vi "Probe.vi"(8 "error in (no error)":errorcluster, 10 "Buffer":u8[](array[numeric]), 11 "Raw Message in":refnum<class "Raw Message.lvclass">) -> (0 "error out":errorcluster, 1 "Valid":bool, 2 "Buffer Count":i32, 3 "Raw Message out":refnum<class "Raw Message.lvclass">)   [LabVIEW 2020, in "Protobuf RAW.lvlib" / "Raw Message.lvclass"]
uses:
  Raw Message.lvclass
  Raw Message.lvclass/Raw Message.ctl
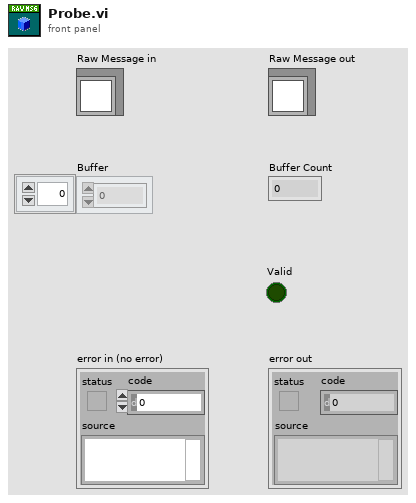
[diagram p1: front panel]
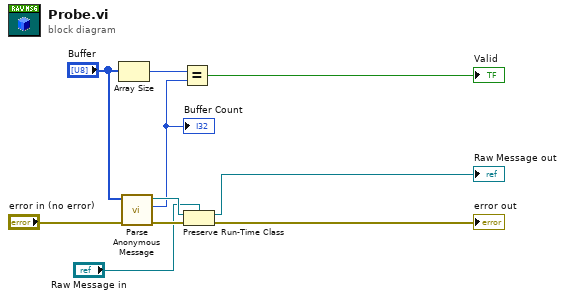
[diagram p0: block diagram]
diagram:
  n1 = Array Size(array="Buffer") -> (size(s)=w4:i32)
  n2 = call "Parse Anonymous Message.vi"("error in (no error)"="error in (no error)", "Buffer"="Buffer") -> ("error out"=w9:errorcluster, "Buffer Length"=w3:i32, "Raw Message"=w7:refnum<class "Raw Message.lvclass">)  [unwired: 7 in]
  "Buffer Count" <- w3
  n3 = Equal?(x=w4, y=w3) -> (x = y?=→"Valid":bool)
  n4 = Preserve Run-Time Class(object in=w7, error in=w9, 2:"Raw Message in") -> (object out=→"Raw Message out":refnum<class "Raw Message.lvclass">, error out=→"error out":errorcluster)
